vi "Get Pattern From String.vi"(8 "error in (no error)":errorcluster {"code" format="%.0x"}, 10 "String Pattern (\"XXXXXXXXXXXXXXXXXX\")":string="XXXXXXXXXXXXXXXXXX", 11 "VISA Resource Name":refnum<visa-resource-name>) -> (0 "error out":errorcluster {"code" format="%.0x"}, 1 "Slope":string, 2 "Edge Source":string, 3 "VISA Resource Name Out":refnum<visa-resource-name>, 5 "Mask":u32, 7 "Pattern Value":u32)   [LabVIEW 2011, in "Agilent 546XX Series.lvlib"]
doc: "This VI returns the numerical value of the string input and correct edge source and slope as defined by the string input."
uses:
  Agilent 546XX Series.lvlib
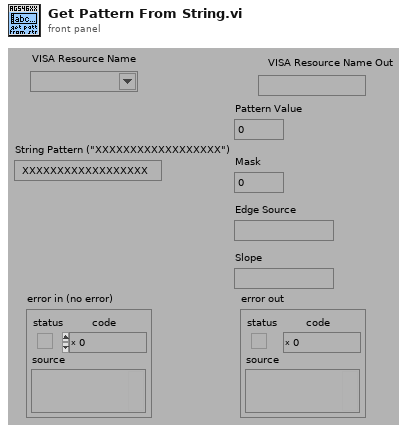
[diagram p1: front panel]
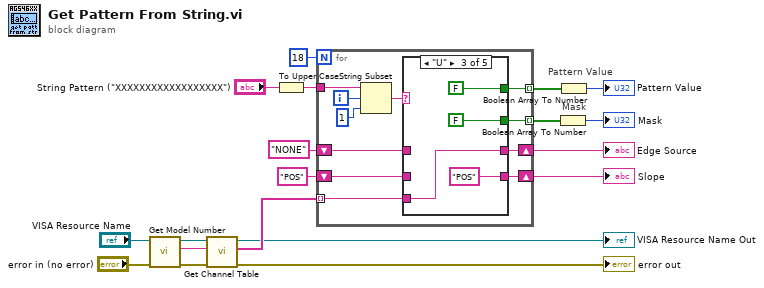
[diagram p0: block diagram]
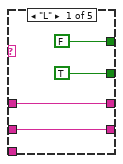
[diagram p2: hidden frame]
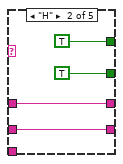
[diagram p3: hidden frame]
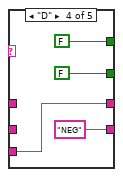
[diagram p4: hidden frame]
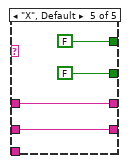
[diagram p5: hidden frame]
diagram:
  # "Pattern Value"
  # "Mask"
  n1 = call "Get Model Number.vi"("error in (no error)"="error in (no error)", "VISA Resource Name"="VISA Resource Name") -> ("error out"=w17:errorcluster, "Model Number"=w16:string, "VISA Resource Name Out"=w18:refnum<visa-resource-name>)  [unwired: 7 in]
  n2 = call "Get Channel Table.vi"("error in (no error)"=w17, "Instrument Model (54621D)"=w16, "VISA Resource Name"=w18) -> ("error out"=→"error out":errorcluster, "Channel Table"=w14:string[], "VISA Resource Name Out"=→"VISA Resource Name Out":refnum<visa-resource-name>)  [unwired: 6 in]
  n3 = To Upper Case(1:"String Pattern (\"XXXXXXXXXXXXXXXXXX\")") -> (0:w9:string)
  n4 = for {
    N: 18 -> [_]
    tunnel: w14 -> [w25] mode=indexing
    shift-right: [w26] -> w1
    shift-left: "POS" -> [w23]
    shift-right: [w24] -> w2
    shift-left: "NONE" ("String") -> [w22]
    tunnel: [w28] -> w13 mode=indexing
    tunnel: [w27] -> w12 mode=indexing
    tunnel: w9 -> [w20]
    i -> [w21]
    n5 = String Subset(string=w20, offset (0)=w21, length (rest)=1 ("length (rest)")) -> (substring=w29:string)
    n6 = case shown="\"U\"" w29 {
      tunnel: [FALSE TRUE FALSE FALSE FALSE] -> w28
      tunnel: [TRUE TRUE FALSE FALSE FALSE] -> w27
      tunnel: [w34 w38 "POS" "NEG" w50] -> w26
      tunnel: w25 -> [_ _ w41 w46 _]
      tunnel: [w33 w37 w41 w46 w49] -> w24
      tunnel: w23 -> [w34 w38 _ _ w50]
      tunnel: w22 -> [w33 w37 _ _ w49]
      frame "L" {
      }
      frame "H" {
      }
      frame "U" {
      }
      frame "D" {
      }
      frame "X", Default {
      }
    }
  }
  "Edge Source" <- w2
  "Slope" <- w1
  n7 = Boolean Array To Number(Boolean array=w12) -> (number=→"Mask":u32)
  n8 = Boolean Array To Number(Boolean array=w13) -> (number=→"Pattern Value":u32)
